vi "WILT Save File.vi"(0 "File Locations":T3[](array[typedef]), 1 "Station Test State Cluster 2":T1, 5 "Array in":T5[](array[typedef]) {"Night Cycle Count" format="%04d"; "Day Cycle Count" format="%04d"}, 7 "File References In":refnum<file>[](array[refnum]), 9 "Fisrt Time Through?":bool[](array[boolean]), 11 "Error In":errorcluster) -> (4 "File Locations Out":T3[](array[typedef]), 6 "First Time Through Out":bool[](array[boolean]), 8 "File References Out":refnum<file>[](array[refnum]), 10 "New File":bool[](array[boolean]), 15 "Error Out":errorcluster)   [LabVIEW 2016]
uses:
  Utility/Save File/File Setup (Public)/Type Definition/Save File DOE File Path Control.ctl
  Utility/Save File/File Setup (Public)/Type Definition/Save File DOE Data Save Filepaths.ctl
  Type Definitions/WILT Dryer.ctl
  Type Definitions/WILT Dryer Details.ctl
  Type Definitions/WILT Agilent Channel Definition.ctl
  Type Definitions/WILT DAQ Data.ctl
  Type Definitions/WILT Station Test State Cluster.ctl
  Type Definitions/WILT Dryer Test State.ctl
  Utility/Save File/File Setup.lvlib
panel:
  # "Day"
  # "Night"
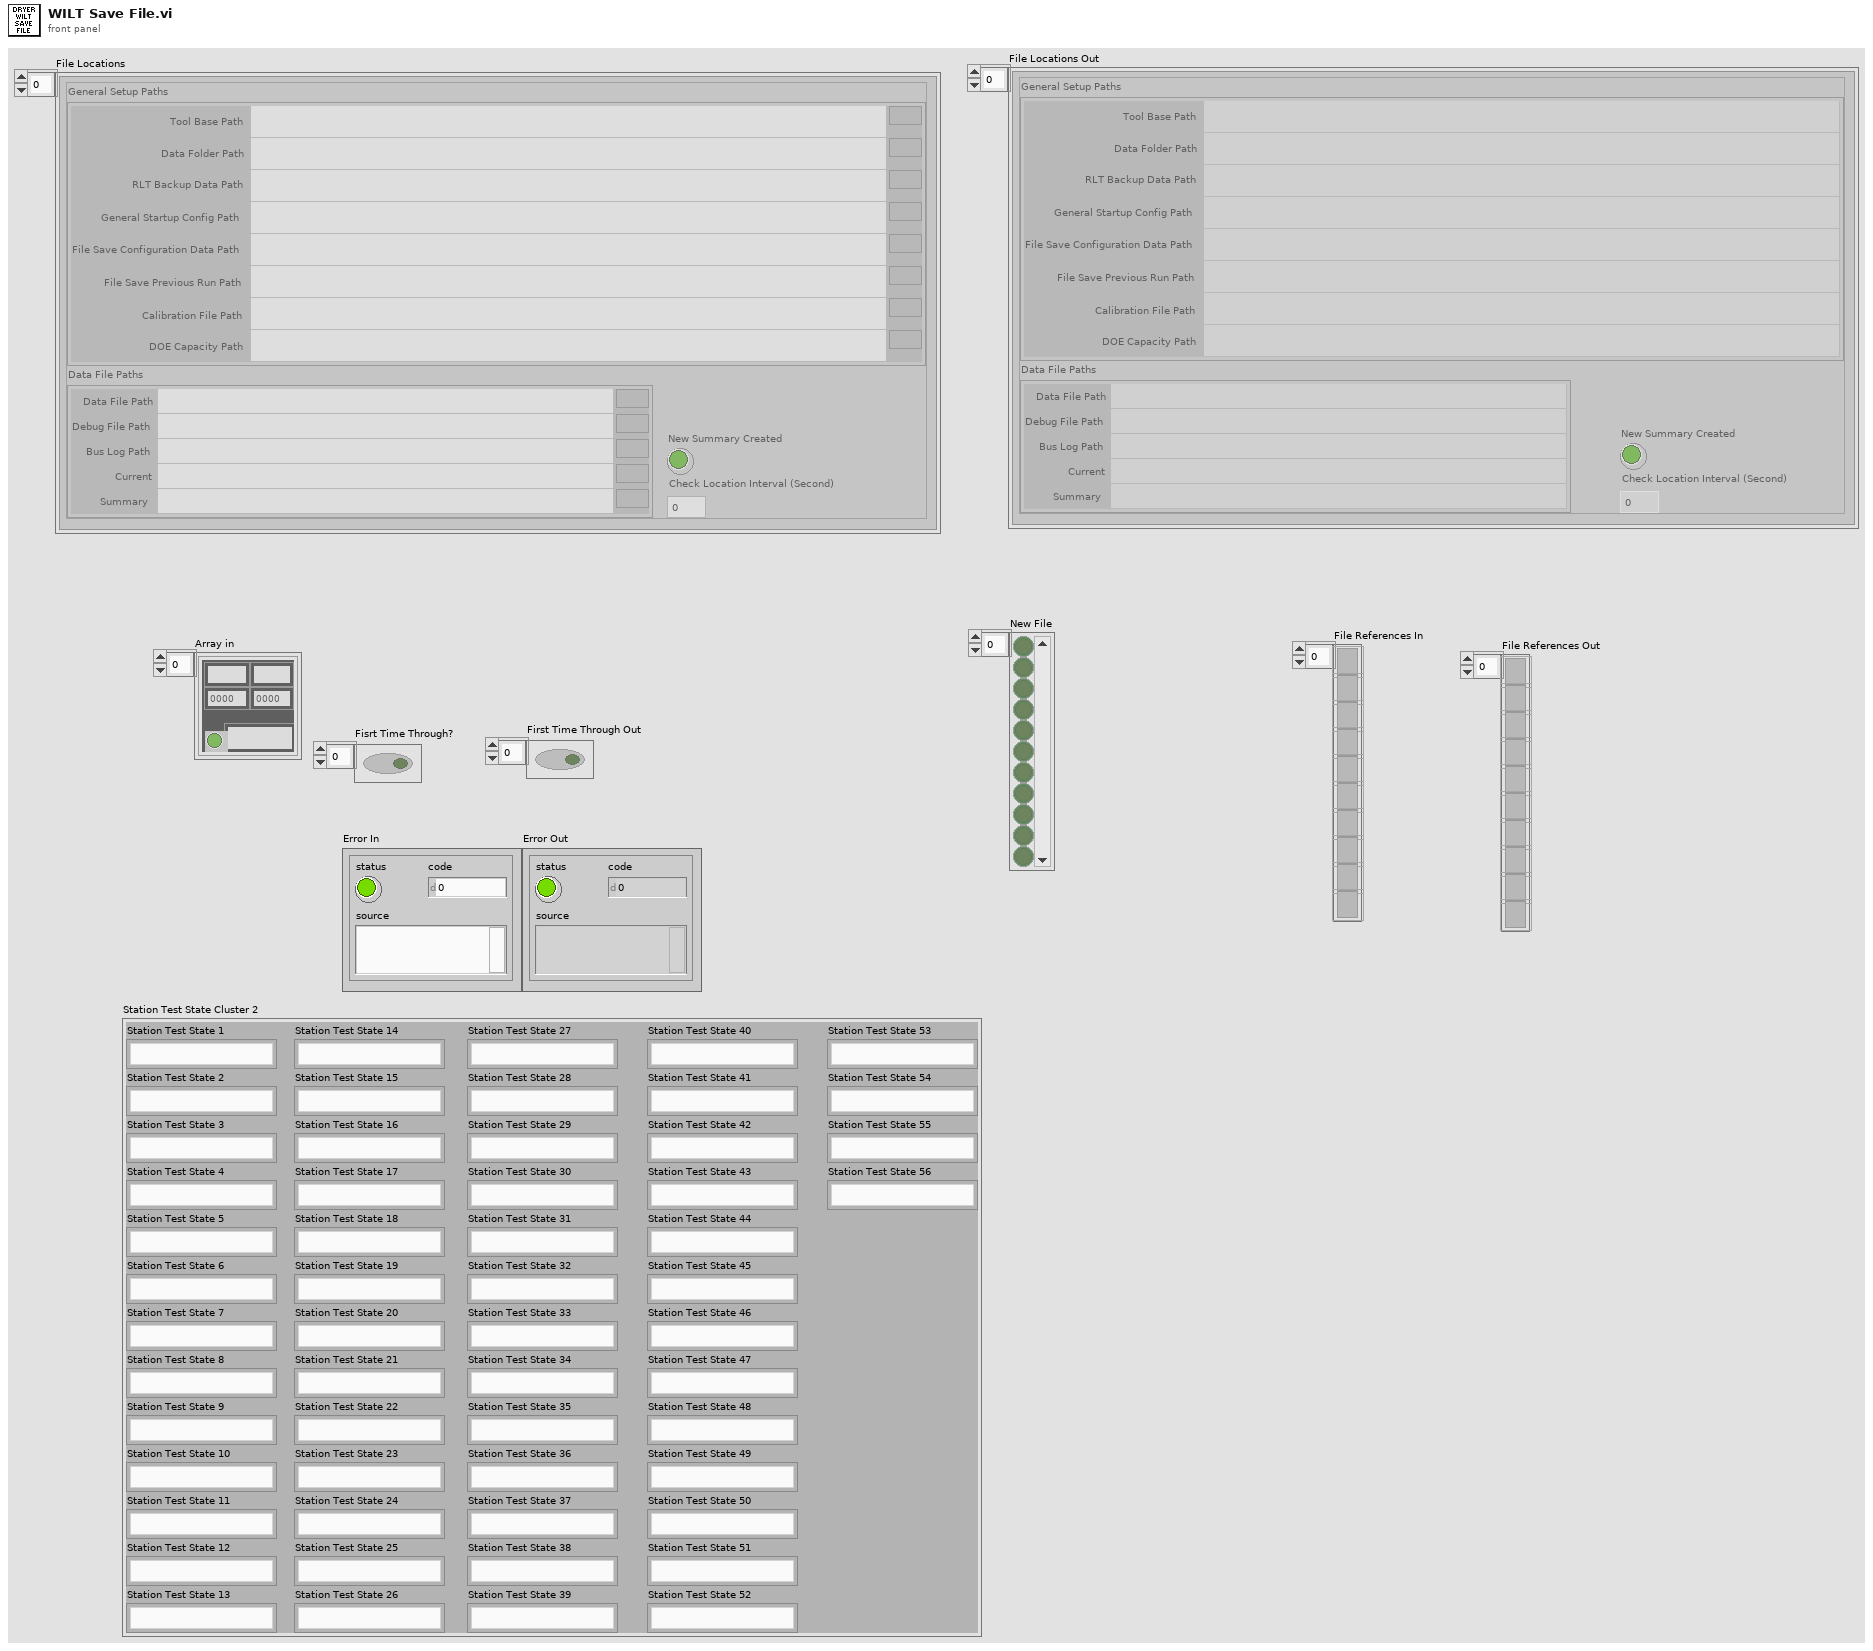
[diagram p1: front panel]
types:
  T1 = typedef "WILT Station Test State Cluster.ctl" = cluster{"Station Test State 1":T2, "Station Test State 2":T2, "Station Test State 3":T2, "Station Test State 4":T2, "Station Test State 5":T2, "Station Test State 6":T2, "Station Test State 7":T2, "Station Test State 8":T2, "Station Test State 9":T2, "Station Test State 10":T2, "Station Test State 11":T2, "Station Test State 12":T2, "Station Test State 13":T2, "Station Test State 14":T2, "Station Test State 15":T2, "Station Test State 16":T2, "Station Test State 17":T2, "Station Test State 18":T2, "Station Test State 19":T2, "Station Test State 20":T2, "Station Test State 21":T2, "Station Test State 22":T2, "Station Test State 23":T2, "Station Test State 24":T2, "Station Test State 25":T2, "Station Test State 26":T2, "Station Test State 27":T2, "Station Test State 28":T2, "Station Test State 29":T2, "Station Test State 30":T2, "Station Test State 31":T2, "Station Test State 32":T2, "Station Test State 33":T2, "Station Test State 34":T2, "Station Test State 35":T2, "Station Test State 36":T2, "Station Test State 37":T2, "Station Test State 38":T2, "Station Test State 39":T2, "Station Test State 40":T2, "Station Test State 41":T2, "Station Test State 42":T2, "Station Test State 43":T2, "Station Test State 44":T2, "Station Test State 45":T2, "Station Test State 46":T2, "Station Test State 47":T2, "Station Test State 48":T2, "Station Test State 49":T2, "Station Test State 50":T2, "Station Test State 51":T2, "Station Test State 52":T2, "Station Test State 53":T2, "Station Test State 54":T2, "Station Test State 55":T2, "Station Test State 56":T2}
  T2 = typedef "WILT Dryer Test State.ctl" = enum16{"No Serial Number", "Waiting for Dryer To Start", "Drying Clothes", "Water Injection 1 (On)", "Water Injection 1 Timer", "Water Injection 1 (Off)", "Pause Dryer", "Sending Start Stop CMD", "Pause Dryer 2", "Sending Start Stop CMD 2", "Drying Clothes 2", "Water Injection 2 (On)", "Water Injection 2 Timer", "Water Injection 2 (Off)", "Drying Clothes 3", "Cooling Down", "Sending Start Stop CMD 3", "Increment Cycle"}
  T3 = typedef "File Setup.lvlib/Save File DOE File Path Control.ctl" = cluster{"General Setup Paths":cluster{"Calibration File Path":path, "DOE Capacity Path":path, "Data Folder Path":path, "RLT Backup Data Path":path, "Tool Base Path":path, "General Startup Config Path":path, "File Save Previous Run Path":path, "File Save Configuration Data Path":path}, "Data File Paths":T4, "New Summary Created":bool, "Check Location Interval (Second)":i32}
  T4 = typedef "File Setup.lvlib/Save File DOE Data Save Filepaths.ctl" = cluster{"Data File Path":path, "Debug File Path":path, "Bus Log Path":path, "Current":path, "Summary":path}
  T5 = typedef "WILT Dryer.ctl" = cluster{"Lab ID":string, "Day Cycle Count":i32, "Station Label":string, "Dryer Details":T6, "Status Color":u32, "Invisible Button":bool, "Night Cycle Count":i32, "Station Index":i32, "Cycle Index":string, "Audit Alert":bool, "Agilent Channel Definition":T7, "DAQ Data":T8}
  T6 = typedef "WILT Dryer Details.ctl" = cluster{"Station":string, "Lab ID":string, "TR Number":string}
  T7 = typedef "WILT Agilent Channel Definition.ctl" = cluster{"Channel":string, "Station":string, "Label":string, "Agilent Station":string, "Data":dbl}
  T8 = typedef "WILT DAQ Data.ctl" = cluster{"L1 Current":dbl, "L2 Current":dbl, "Temperature  Deg F (TC)":dbl, "Volts":dbl, "Volts (208)":dbl, "SW (208)":dbl}
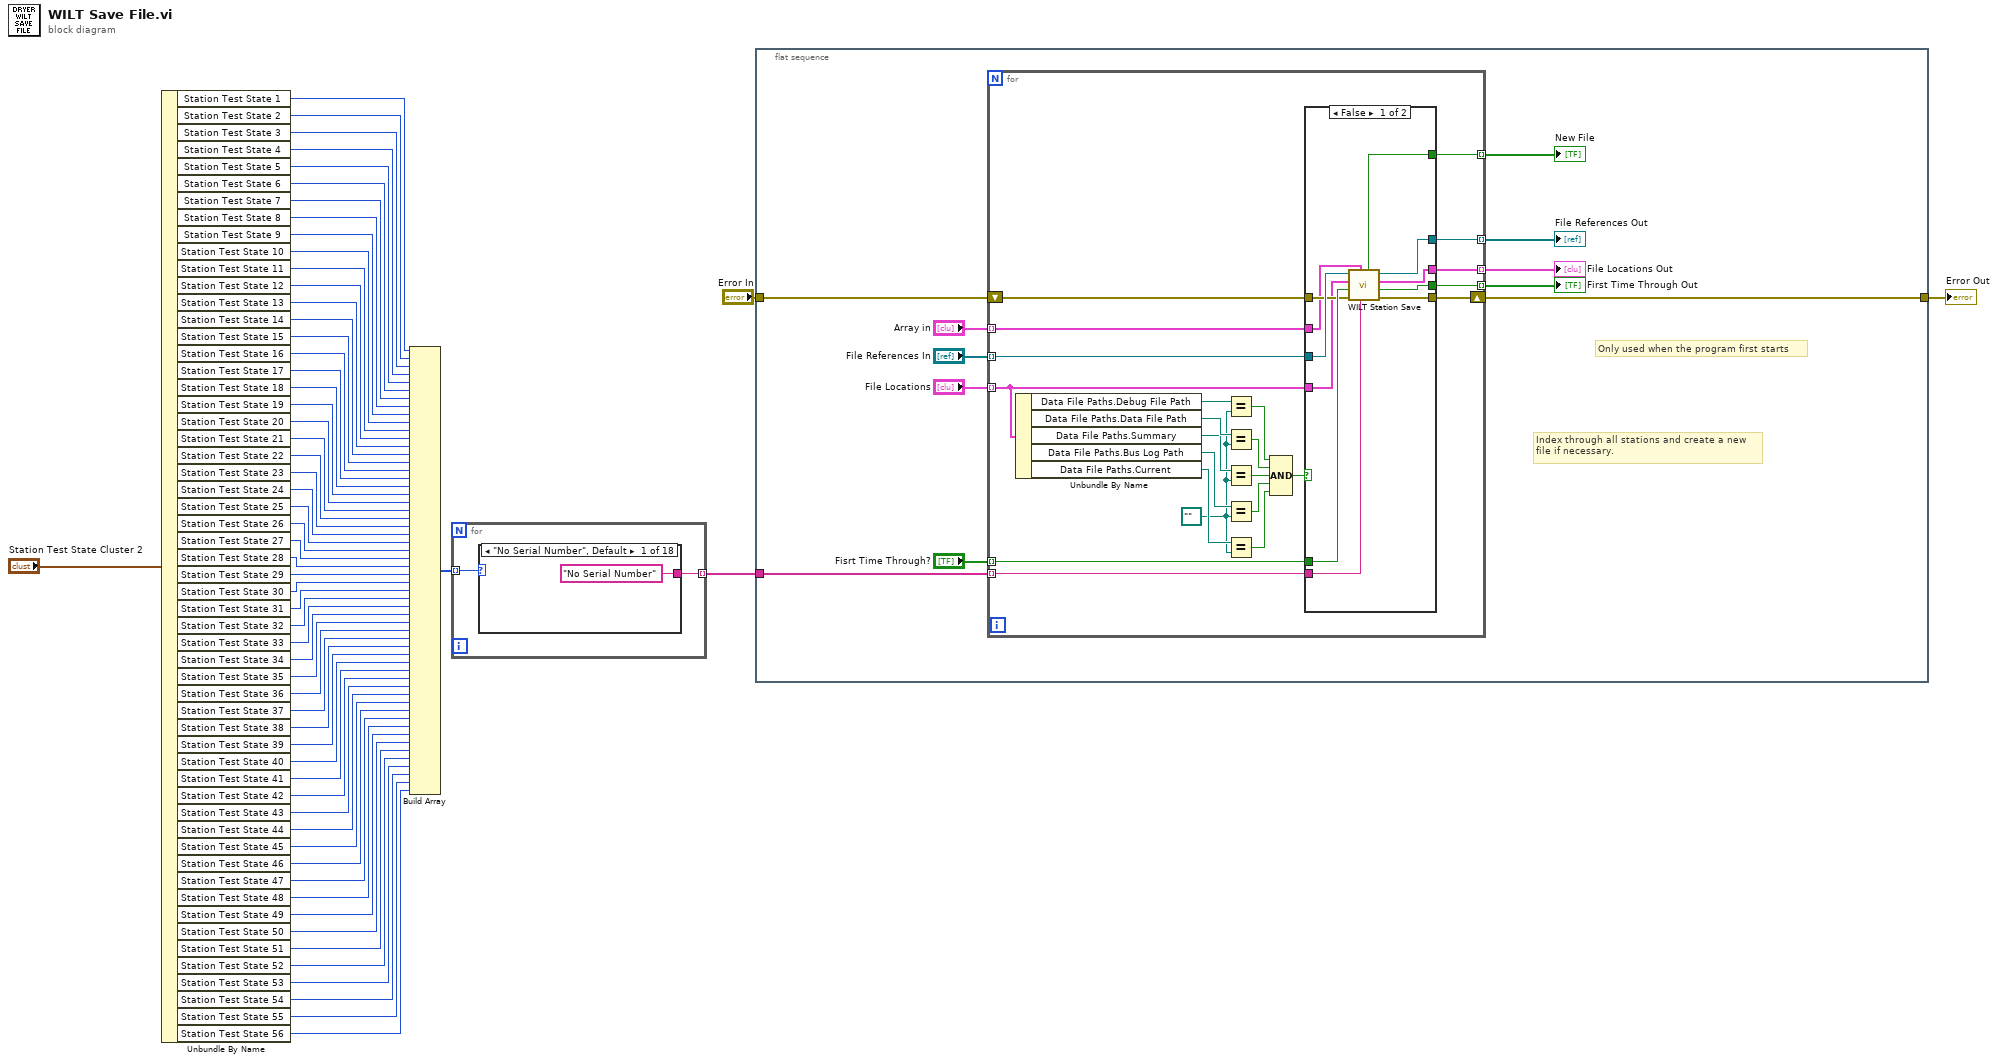
[diagram p0: block diagram]
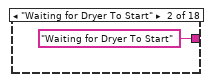
[diagram p2: hidden frame]
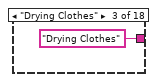
[diagram p3: hidden frame]
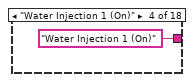
[diagram p4: hidden frame]
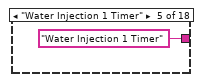
[diagram p5: hidden frame]
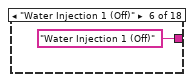
[diagram p6: hidden frame]
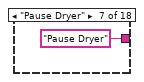
[diagram p7: hidden frame]
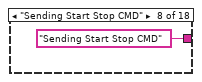
[diagram p8: hidden frame]
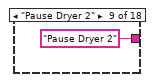
[diagram p9: hidden frame]
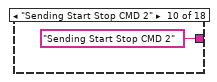
[diagram p10: hidden frame]
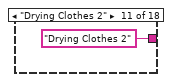
[diagram p11: hidden frame]
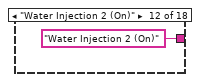
[diagram p12: hidden frame]
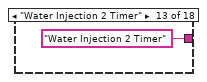
[diagram p13: hidden frame]
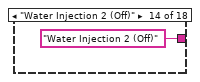
[diagram p14: hidden frame]
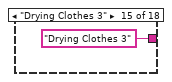
[diagram p15: hidden frame]
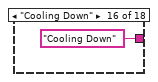
[diagram p16: hidden frame]
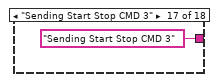
[diagram p17: hidden frame]
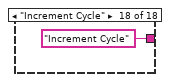
[diagram p18: hidden frame]
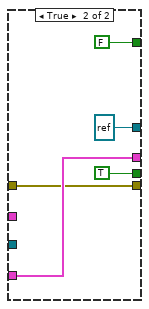
[diagram p19: hidden frame]
diagram:
  n1 = Unbundle By Name("Station Test State Cluster 2") -> ("Station Test State 1"=w58:T2, "Station Test State 2"=w57:T2, "Station Test State 3"=w56:T2, "Station Test State 4"=w55:T2, "Station Test State 5"=w54:T2, "Station Test State 6"=w53:T2, "Station Test State 7"=w52:T2, "Station Test State 8"=w51:T2, "Station Test State 9"=w50:T2, "Station Test State 10"=w49:T2, "Station Test State 11"=w48:T2, "Station Test State 12"=w47:T2, "Station Test State 13"=w46:T2, "Station Test State 14"=w45:T2, "Station Test State 15"=w44:T2, "Station Test State 16"=w43:T2, "Station Test State 17"=w42:T2, "Station Test State 18"=w41:T2, "Station Test State 19"=w40:T2, "Station Test State 20"=w39:T2, "Station Test State 21"=w38:T2, "Station Test State 22"=w37:T2, "Station Test State 23"=w36:T2, "Station Test State 24"=w35:T2, "Station Test State 25"=w34:T2, "Station Test State 26"=w33:T2, "Station Test State 27"=w32:T2, "Station Test State 28"=w31:T2, "Station Test State 29"=w30:T2, "Station Test State 30"=w29:T2, "Station Test State 31"=w28:T2, "Station Test State 32"=w27:T2, "Station Test State 33"=w26:T2, "Station Test State 34"=w25:T2, "Station Test State 35"=w24:T2, "Station Test State 36"=w23:T2, "Station Test State 37"=w22:T2, "Station Test State 38"=w21:T2, "Station Test State 39"=w20:T2, "Station Test State 40"=w19:T2, "Station Test State 41"=w18:T2, "Station Test State 42"=w17:T2, "Station Test State 43"=w16:T2, "Station Test State 44"=w15:T2, "Station Test State 45"=w14:T2, "Station Test State 46"=w13:T2, "Station Test State 47"=w12:T2, "Station Test State 48"=w11:T2, "Station Test State 49"=w10:T2, "Station Test State 50"=w9:T2, "Station Test State 51"=w8:T2, "Station Test State 52"=w7:T2, "Station Test State 53"=w6:T2, "Station Test State 54"=w5:T2, "Station Test State 55"=w4:T2, "Station Test State 56"=w3:T2)
  n2 = Build Array(w58, w57, w56, w55, w54, w53, w52, w51, w50, w49, w48, w47, w46, w45, w44, w43, w42, w41, w40, w39, w38, w37, w36, w35, w34, w33, w32, w31, w30, w29, w28, w27, w26, w25, w24, w23, w22, w21, w20, w19, w18, w17, w16, w15, w14, w13, w12, w11, w10, w9, w8, w7, w6, w5, w4, w3) -> (w2:T2[])
  n3 = for {
    tunnel: w2 -> [w63] mode=indexing
    tunnel: [w62] -> w1 mode=indexing
    n4 = case shown="\"No Serial Number\", Default" w63 {
      tunnel: ["No Serial Number" "Waiting for Dryer To Start" "Drying Clothes" "Water Injection 1 (On)" "Water Injection 1 Timer" "Water Injection 1 (Off)" "Pause Dryer" "Sending Start Stop CMD" "Pause Dryer 2" "Sending Start Stop CMD 2" "Drying Clothes 2" "Water Injection 2 (On)" "Water Injection 2 Timer" "Water Injection 2 (Off)" "Drying Clothes 3" "Cooling Down" "Sending Start Stop CMD 3" "Increment Cycle"] -> w62
      frame "No Serial Number", Default {
      }
      frame "Waiting for Dryer To Start" {
      }
      frame "Drying Clothes" {
      }
      frame "Water Injection 1 (On)" {
      }
      frame "Water Injection 1 Timer" {
      }
      frame "Water Injection 1 (Off)" {
      }
      frame "Pause Dryer" {
      }
      frame "Sending Start Stop CMD" {
      }
      frame "Pause Dryer 2" {
      }
      frame "Sending Start Stop CMD 2" {
      }
      frame "Drying Clothes 2" {
      }
      frame "Water Injection 2 (On)" {
      }
      frame "Water Injection 2 Timer" {
      }
      frame "Water Injection 2 (Off)" {
      }
      frame "Drying Clothes 3" {
      }
      frame "Cooling Down" {
      }
      frame "Sending Start Stop CMD 3" {
      }
      frame "Increment Cycle" {
      }
    }
  }
  n5 = flat-sequence {
    tunnel: "Error In" -> [w84]
    tunnel: [w83] -> w60
    tunnel: w1 -> [w82]
    frame #0 {
      # "Only used when the program first starts"
      # "Index through all stations and create a new\nfile if necessary."
      n6 = for {
        tunnel: "File Locations" -> [w106] mode=indexing
        tunnel: [w112] -> w90 mode=indexing
        tunnel: "Array in" -> [w107] mode=indexing
        tunnel: "Fisrt Time Through?" -> [w115] mode=indexing
        tunnel: [w114] -> w89 mode=indexing
        tunnel: [w113] -> w87 mode=indexing
        tunnel: [w111] -> w86 mode=indexing
        tunnel: "File References In" -> [w110] mode=indexing
        shift-right: [w108] -> w83
        shift-left: w84 -> [w109]
        tunnel: w82 -> [w93] mode=indexing
        w100 = path "" ("Log Debug File")
        n7 = Unbundle By Name(w106) -> ("Data File Paths.Debug File Path"=w105:path, "Data File Paths.Data File Path"=w104:path, "Data File Paths.Summary"=w103:path, "Data File Paths.Bus Log Path"=w102:path, "Data File Paths.Current"=w101:path)
        n8 = Equal?(x=w105, y=w100) -> (x = y?=w99:bool)
        n9 = Equal?(x=w104, y=w100) -> (x = y?=w98:bool)
        n10 = Equal?(x=w103, y=w100) -> (x = y?=w97:bool)
        n11 = Equal?(x=w102, y=w100) -> (x = y?=w96:bool)
        n12 = Equal?(x=w101, y=w100) -> (x = y?=w95:bool)
        n13 = Compound Arithmetic op=AND(w99, w98, w97, w96, w95) -> (w94:bool)
        n14 = case shown="False" w94 {
          tunnel: w115 -> [w126 _]
          tunnel: [w125 TRUE ("First Time Through Out")] -> w114
          tunnel: [w124 FALSE ("New File?")] -> w113
          tunnel: [w123 w131] -> w112
          tunnel: [w122 refnum<file> refnum ("Byte Stream File out")] -> w111
          tunnel: w110 -> [w121 _]
          tunnel: w109 -> [w120 w127]
          tunnel: [w119 w127] -> w108
          tunnel: w107 -> [w118 _]
          tunnel: w106 -> [w117 w131]
          tunnel: w93 -> [w116 _]
          frame False {
            n15 = call "WILT Station Save.vi"("Test Station State"=w116, "Dryer 14"=w118, "error in (no error)"=w120, "First Time Through?"=w126, "File Locations A"=w117, "Byte Stream File in"=w121) -> ("error out"=w119:errorcluster, "First Time Through Out"=w125:bool, "File Path Output New out"=w123:T3, "Byte Stream File out"=w122:refnum<file>, "New File?"=w124:bool)  [unwired: 1 in]
          }
          frame True {
          }
        }
      }
      "File Locations Out" <- w90
      "First Time Through Out" <- w89
      "New File" <- w87
      "File References Out" <- w86
    }
  }
  "Error Out" <- w60
